vi "Select axes.vi"(0 "Cluster":T1, 3 "output array":string[][](array[string])) -> (4 "index of y":i32, 5 "XY Graph":cluster{dbl[], dbl[]}[](graph), 7 "index of x":i32=1)   [LabVIEW 2013]
panel:
  out "Array":bool[](array[boolean])
  out "appended array 2":string[][](array[string])
  out "appended array":string[][](array[string])
  out "index of y 2":i32
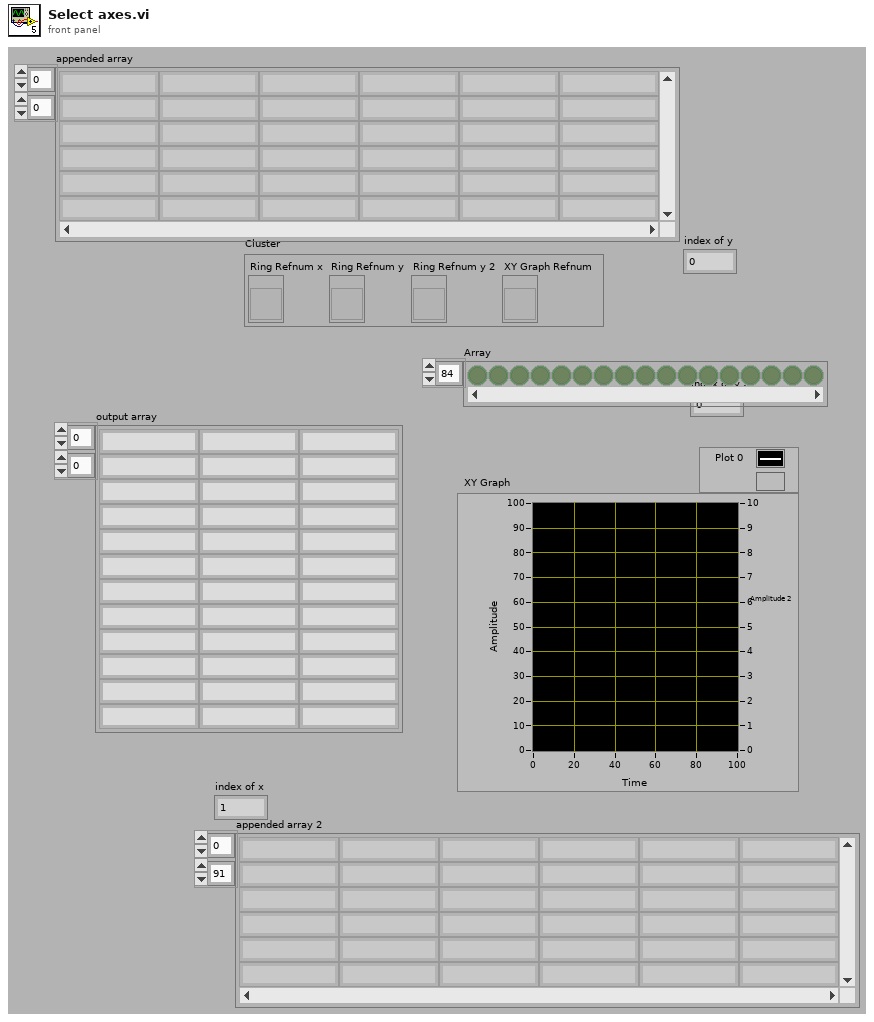
[diagram p1: front panel]
types:
  T1 = cluster{"Ring Refnum x":refnum<vi>, "Ring Refnum y":refnum<vi>, "Ring Refnum y 2":refnum<vi>, "XY Graph Refnum":refnum<vi>}
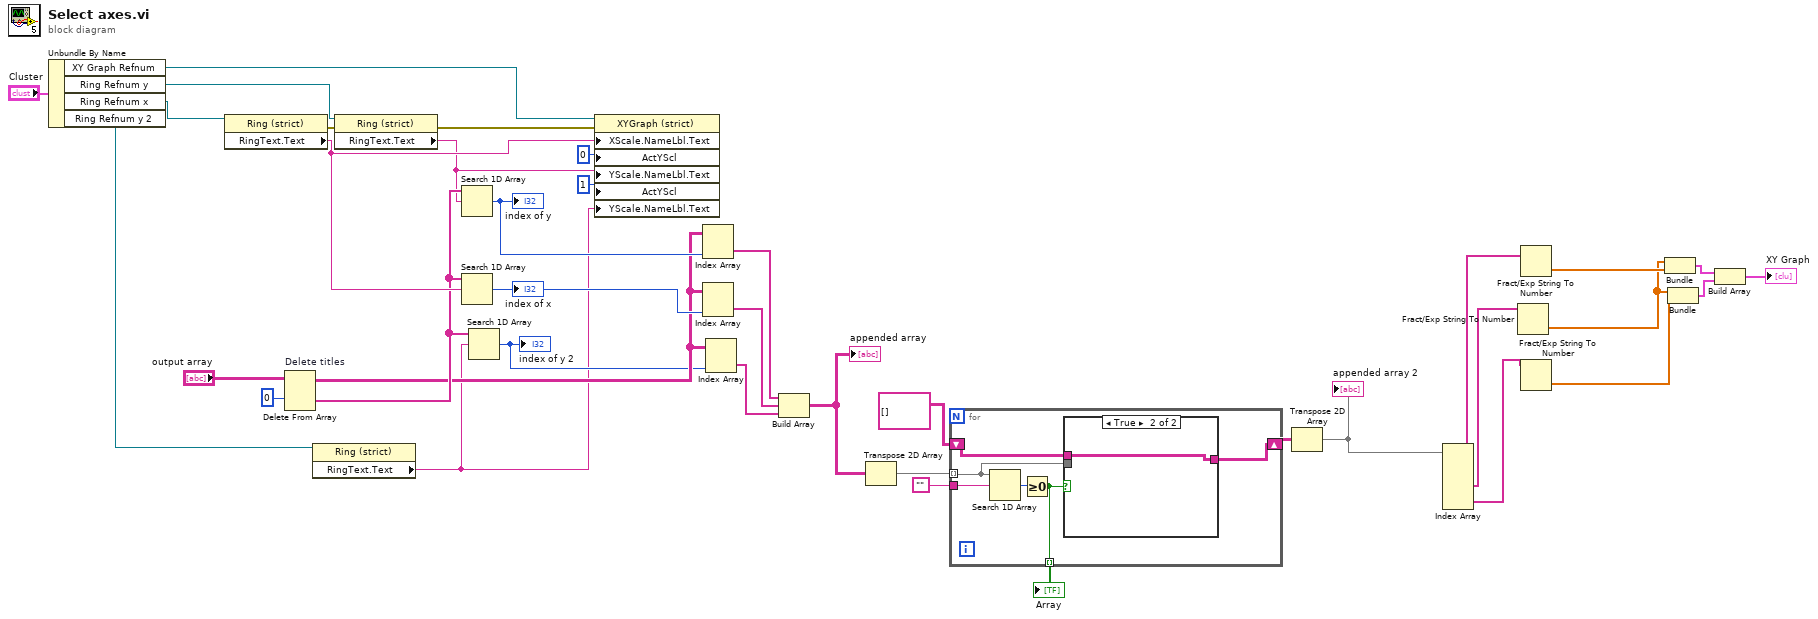
[diagram p0: block diagram]
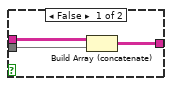
[diagram p2: hidden frame]
diagram:
  n1 = Unbundle By Name("Cluster") -> ("XY Graph Refnum"=w15:refnum<vi>, "Ring Refnum y"=w16:refnum<vi>, "Ring Refnum x"=w17:refnum<vi>, "Ring Refnum y 2"=w14:refnum<vi>)
  n2 = property on="Property Node" class="Ring (strict)"(reference=w17) -> (error out=w37:errorcluster, "RingText.Text"=w36:string)  [unwired: 1 in, 1 out]
  n3 = Delete From Array "Delete titles"(array="output array", index (row)=0) -> (deleted portion=w30:string[], array with subset deleted=w27:string[][])  [unwired: 2 in]
  n4 = property on="Property Node" class="Ring (strict)"(reference=w14) -> ("RingText.Text"=w19:string)  [unwired: 1 in, 2 out]
  n5 = property on="Property Node" class="Ring (strict)"(reference=w16, error in=w37) -> (error out=w38:errorcluster, "RingText.Text"=w22:string)  [unwired: 1 out]
  n6 = Search 1D Array(1D array=w30, element=w22) -> (index of element=w34:i32)  [unwired: 1 in]
  "index of y" <- w34
  n7 = Search 1D Array(1D array=w30, element=w36) -> (index of element=w33:i32)  [unwired: 1 in]
  "index of x" <- w33
  n8 = Search 1D Array(1D array=w30, element=w19) -> (index of element=w26:i32)  [unwired: 1 in]
  "index of y 2" <- w26
  n9 = property on="Property Node" class="XYGraph (strict)"(reference=w15, error in=w38, "XScale.NameLbl.Text"=w36, "ActYScl"=0 ("Active Y Scale"), "YScale.NameLbl.Text"=w22, "ActYScl"=1 ("Active Y Scale"), "YScale.NameLbl.Text"=w19) -> ()  [unwired: 2 out]
  n10 = Index Array(array=w27, index (col)=w34) -> (element=w13:string[])  [unwired: 1 in]
  n11 = Index Array(array=w27, index (col)=w33) -> (element=w12:string[])  [unwired: 1 in]
  n12 = Index Array(array=w27, index (col)=w26) -> (element=w11:string[])  [unwired: 1 in]
  n13 = Build Array(w13, w12, w11) -> (w5:string[][])
  "appended array" <- w5
  n14 = Transpose 2D Array(2D array=w5) -> (transposed array=w9:string[][])
  n15 = for {
    tunnel: w9 -> [w40] mode=indexing
    tunnel: "" -> [w44]
    shift-right: [w41] -> w8
    shift-left: string[][] [] -> [w42]
    tunnel: [w39] -> w6 mode=indexing
    n16 = Search 1D Array(1D array=w40, element=w44) -> (index of element=w43:i32)  [unwired: 1 in]
    n17 = Greater Or Equal To 0?(x=w43) -> (x >= 0?=w39:bool)
    n18 = case shown="True" w39 {
      tunnel: w42 -> [w47 w48]
      tunnel: [w46 w48] -> w41
      tunnel: w40 -> [w45 _]
      frame False {
        n19 = Build Array (concatenate)(w47, w45) -> (w46:string[][])
      }
      frame True {
      }
    }
  }
  "Array" <- w6
  n20 = Transpose 2D Array(2D array=w8) -> (transposed array=w4:string[][])
  "appended array 2" <- w4
  n21 = Index Array(array=w4) -> (element #1=w3:string[], element #2=w2:string[], element #3=w1:string[])  [unwired: 6 in]
  n22 = Fract/Exp String To Number(string=w2) -> (number=w29:dbl[])  [unwired: 3 in, 1 out]
  n23 = Fract/Exp String To Number(string=w3) -> (number=w35:dbl[])  [unwired: 3 in, 1 out]
  n24 = Fract/Exp String To Number(string=w1) -> (number=w28:dbl[])  [unwired: 3 in, 1 out]
  n25 = Bundle(w29, w35) -> (w25:cluster{dbl[], dbl[]})  [unwired: 1 in]
  n26 = Bundle(w29, w28) -> (w24:cluster{dbl[], dbl[]})  [unwired: 1 in]
  n27 = Build Array(w25, w24) -> (→"XY Graph":cluster{dbl[], dbl[]}[])
